vi "Double FFT Mesurament (Max Bin detection & Init Mem) test.vi"   [LabVIEW 2014]
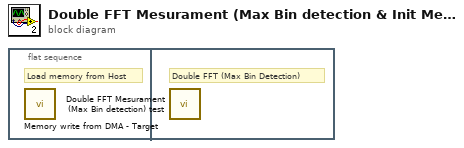
[diagram p0: block diagram]
diagram:
  n1 = flat-sequence {
    frame #0 {
      # "Load memory from Host"
      n2 = call "Memory write from DMA - Target.vi"() -> ()  [unwired: 12 in]
    }
    frame #1 {
      # "Double FFT (Max Bin Detection)"
      n3 = call "Double FFT Mesurament (Max Bin detection) test.vi"() -> ()  [unwired: 12 in]
    }
  }
